vi "GetTelemetryUpdateDataSGLConstant.vi"() -> (3 "TelemetryUpdateDataSGL":T1={"Mode"=enum."=", "Field"=enum."InclinometerErrorCode", "Data"=0.0})   [LabVIEW 2016]
uses:
  TelemetryUpdateDataSGL.ctl
  TelemetryUpdateModes.ctl
  TelemetryFields.ctl
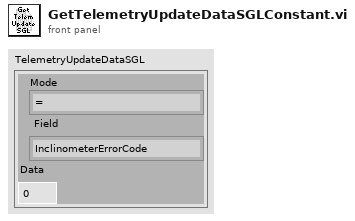
[diagram p1: front panel]
types:
  T1 = typedef "TelemetryUpdateDataSGL.ctl" = cluster{"Mode":T2, "Field":T3, "Data":sgl}
  T2 = typedef "TelemetryUpdateModes.ctl" = enum8{"=", "+", "-", "|"}
  T3 = typedef "TelemetryFields.ctl" = enum16{"None", "InclinometerTxBytes", "InclinometerRxBytes", "InclinometerTxFrames", "InclinometerRxFrames", "InclinometerErrorTimestamp", "InclinometerErrorCode", "InclinometerSampleTimestamp", "InclinometerRawAngle", "InclinometerZenithAngle", "DisplacementTxBytes", "DisplacementRxBytes", "DisplacementTxFrames", "DisplacementRxFrames", "DisplacementErrorTimestamp", "DisplacementErrorCode", "DisplacementSampleTimestamp", "DisplacementRaw1", "DisplacementRaw2", "DisplacementRaw3", "DisplacementRaw4", "DisplacementRaw5", "DisplacementRaw6", "DisplacementRaw7", "DisplacementRaw8", "DisplacementEng1", "DisplacementEng2", "DisplacementEng3", "DisplacementEng4", "DisplacementEng5", "DisplacementEng6", "DisplacementEng7", "DisplacementEng8", "DisplacementPositionX", "DisplacementPositionY", "DisplacementPositionZ", "DisplacementRotationX", "DisplacementRotationY", "DisplacementRotationZ", "AccelerometerSampleCount", "AccelerometerSampleTimestamp", "AccelerometerRaw1", "AccelerometerRaw2", "AccelerometerRaw3", "AccelerometerRaw4", "AccelerometerRaw5", "AccelerometerRaw6", "AccelerometerRaw7", "AccelerometerRaw8", "AccelerometerEng1", "AccelerometerEng2", "AccelerometerEng3", "AccelerometerEng4", "AccelerometerEng5", "AccelerometerEng6", "AccelerometerEng7", "AccelerometerEng8", "AngularAccelerationX", "AngularAccelerationY", "AngularAccelerationZ", "GyroTxBytes", "GyroRxBytes", "GyroTxFrames", "GyroRxFrames", "GyroErrorTimestamp", "GyroErrorCode", "GyroSampleTimestamp", "GyroX", "GyroY", "GyroZ", "GyroStatus", "GyroSequenceNumber", "GyroTemperature", "GyroBITTimestamp", "GyroBIT0", "GyroBIT1", "GyroBIT2", "GyroBIT3", "GyroBIT4", "GyroBIT5", "GyroBIT6", "GyroBIT7"}
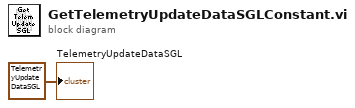
[diagram p0: block diagram]
diagram:
  "TelemetryUpdateDataSGL" <- T1 {"Mode"=enum."=", "Field"=enum."InclinometerErrorCode", "Data"=0.0} ("TelemetryUpdateDataSGL")
